vi "getTemperature.vi"(6 "Channel":i32, 8 "error in (no error)":errorcluster, 11 "instrument.PPMS":refnum<class "instrument.PPMS.lvclass">) -> (0 "error out":errorcluster, 1 "Status":string, 2 "Temperature (K)":dbl, 3 "instrument.PPMS out":refnum<class "instrument.PPMS.lvclass">, 4 "Finished?":bool)   [LabVIEW 2019, in "instrument.PPMS.lvclass"]
uses:
  instrument.PPMS.lvclass
  C:/Program Files (x86)/National Instruments/LabVIEW 2019/user.lib/LevyLab/Instrument Framework/Instrument/Instrument.lvclass
  <vilib>/AdvancedString/1D String Array to Delimited String.vi
  23df749e-c1f3-4610-888a-6b8f4af7e3d0.vi/2ff18fbe-3cd5-4aa6-be5b-70698d1896b0.vi
  <vilib>/Utility/Data Type/Get Type Information.vi
  <vilib>/Utility/Data Type/Get Numeric Information.vi
  <userlib>/_OpenG.lib/lvdata/lvdata.llb/Unwrap VVariant__ogtk.vi
  <userlib>/LevyLab/Instrument Framework/Instrument/API/Remote Client.vi
  <vilib>/Utility/error.llb/Error Cluster From Error Code.vi
  <userlib>/LevyLab/Instrument Framework/Instrument Types/Cryostat/Instrument.Cryostat.lvclass
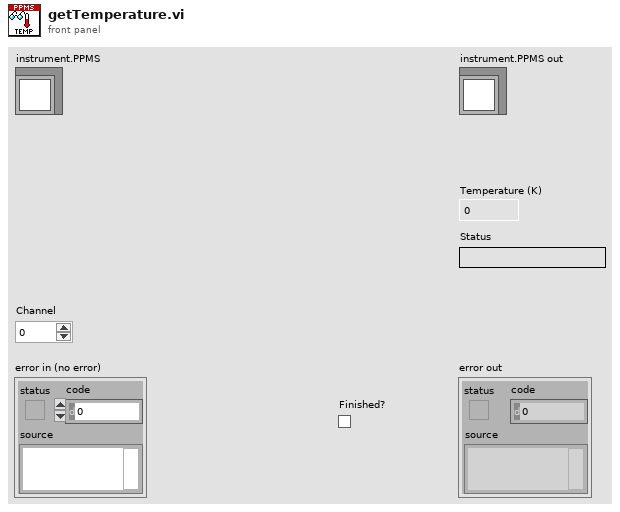
[diagram p1: front panel]
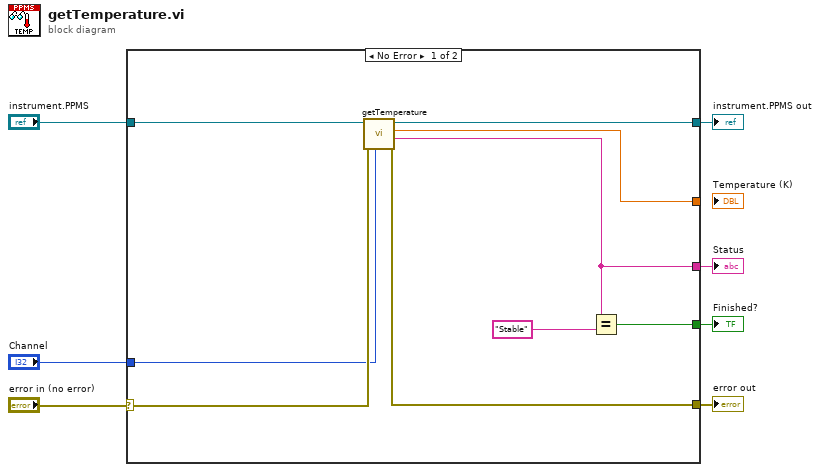
[diagram p0: block diagram]
diagram:
  n1 = case shown="No Error" "error in (no error)" {
    selector: "error in (no error)" -> [w12 w18]
    tunnel: [w10 _] -> _
    tunnel: [w11 w18] -> w7
    tunnel: [w13 w17] -> w6
    tunnel: "instrument.PPMS" -> [w16 w17]
    tunnel: [w14 _] -> w3
    tunnel: [w9 _] -> w2
    tunnel: "Channel" -> [w8 _]
    frame No Error {
      n2 = call-parent "getTemperature.vi"("Channel"=w8, "error in (no error)"=w12, "Instrument.Cryostat in"=w16) -> ("error out"=w11:errorcluster, "Status"=w9:string, "Temperature (K)"=w10:dbl, "Instrument.Cryostat out"=w13:refnum<class "instrument.PPMS.lvclass">)  [unwired: 4 in, 1 out]
      n3 = Equal?(x=w9, y="Stable" ("Temperature Status")) -> (x = y?=w14:bool)
    }
    frame Error {
    }
  }
  "error out" <- w7
  "instrument.PPMS out" <- w6
  "Status" <- w2
  "Finished?" <- w3
